vi "Generate Comments.vi"(7 "error in (no error)":errorcluster, 10 "AFM Control":refnum<class "AFM Control.lvclass">) -> (0 "error out":errorcluster, 2 "Comments":string, 3 "AFM Control out":refnum<class "AFM Control.lvclass">)   [LabVIEW 2020, in "AFM Control.lvclass"]
uses:
  AFM Control.lvclass
  AFM Control.lvclass/AFM Control.ctl
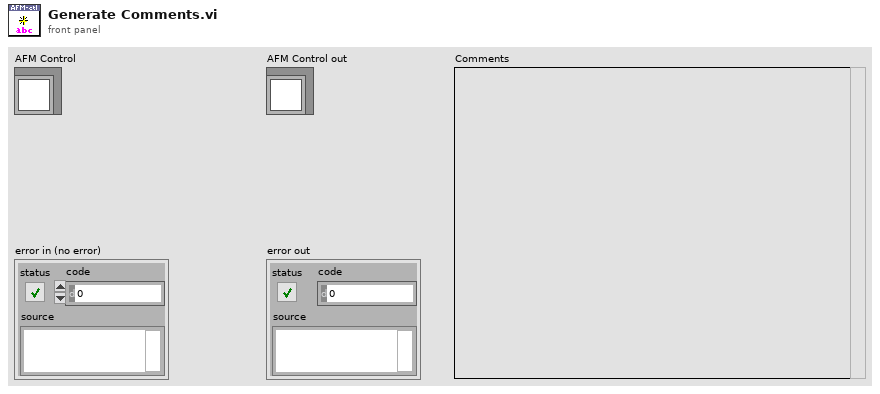
[diagram p1: front panel]
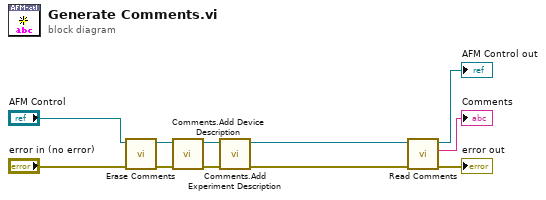
[diagram p0: block diagram]
diagram:
  n1 = call "Erase Comments.vi"("error in (no error)"="error in (no error)", "AFM Control"="AFM Control") -> ("error out"=w3:errorcluster, "AFM Control out"=w5:refnum<class "AFM Control.lvclass">)  [unwired: 8 in]
  n2 = call "Comments.Add Device Description.vi"("error in (no error)"=w3, "AFM Control"=w5) -> ("error out"=w10:errorcluster, "AFM Control out"=w11:refnum<class "AFM Control.lvclass">)  [unwired: 8 in]
  n3 = call "Comments.Add Experiment Description.vi"("error in (no error)"=w10, "AFM Control"=w11) -> ("error out"=w1:errorcluster, "AFM Control out"=w2:refnum<class "AFM Control.lvclass">)  [unwired: 7 in]
  n4 = call "Read Comments.vi"("error in (no error)"=w1, "AFM Control"=w2) -> ("error out"=→"error out":errorcluster, "Comments"=→"Comments":string, "AFM Control out"=→"AFM Control out":refnum<class "AFM Control.lvclass">)  [unwired: 7 in]
